vi "Resize.vi"(1 "Draw Area Size":T1, 2 "image data":T2) -> (0 "Numeric Control":dbl)   [LabVIEW 2014]
doc: "Resizes the given image to fit the picture control that contains it. The zoom factor for the control is returned"
uses:
  <vilib>/picture/picture.llb/imagedata.ctl
  <vilib>/Utility/miscctls.llb/LVBoundsTypeDef.ctl
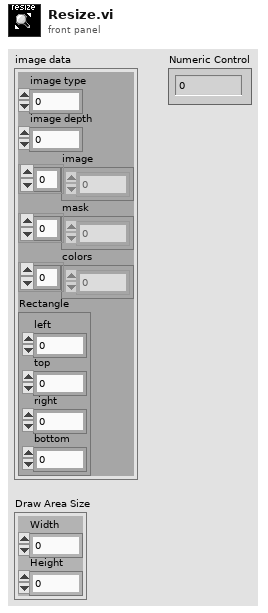
[diagram p1: front panel]
types:
  T1 = typedef "LVBoundsTypeDef.ctl" = cluster{"Width":u32, "Height":u32}
  T2 = typedef "imagedata.ctl" = cluster{"image type":i32, "image depth":i32, "image":u8[], "mask":u8[], "colors":u32[], "Rectangle":cluster{"left":i16, "top":i16, "right":i16, "bottom":i16}}
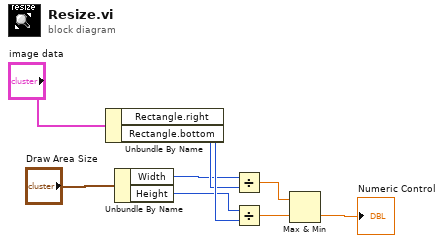
[diagram p0: block diagram]
diagram:
  n1 = Unbundle By Name("image data") -> ("Rectangle.right"=w7:i16, "Rectangle.bottom"=w8:i16)
  n2 = Unbundle By Name("Draw Area Size") -> ("Width"=w2:u32, "Height"=w3:u32)
  n3 = Divide(x=w2, y=w7) -> (x/y=w4:dbl)
  n4 = Divide(x=w3, y=w8) -> (x/y=w5:dbl)
  n5 = Max & Min(x=w4, y=w5) -> (min(x,y)=→"Numeric Control":dbl)  [unwired: 1 out]
